vi "NumToString.vi"(0 "Numeric":dbl, 5 "error in (no error)":errorcluster) -> (14 "String":string, 19 "error out":errorcluster)   [LabVIEW 2017, in "TestLibrary.lvlib" / "GSharpCls.lvclass"]
uses:
  GSharpCls.lvclass
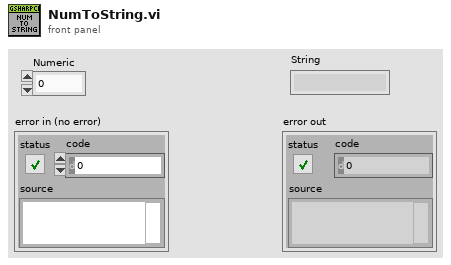
[diagram p1: front panel]
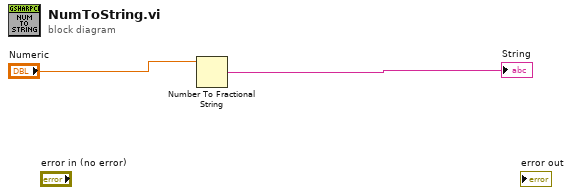
[diagram p0: block diagram]
diagram:
  n1 = Number To Fractional String(number="Numeric") -> (F-format string=→"String":string)  [unwired: 3 in]
